vi "Read Stamping.vi"(8 "error in (no error)":errorcluster, 11 "Gluing Procedure in":refnum<class "Gluing Procedure.lvclass">) -> (0 "error out":errorcluster, 2 "Stamping":T1, 3 "Gluing Procedure out":refnum<class "Gluing Procedure.lvclass">)   [LabVIEW 2017, in "Gluing Procedure.lvclass"]
uses:
  Gluing Procedure.lvclass
  Type Definitions/Stamping.ctl
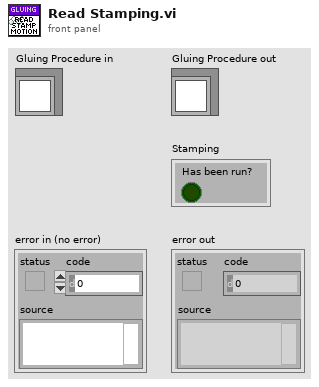
[diagram p1: front panel]
types:
  T1 = typedef "Stamping.ctl" = cluster{"Has been run?":bool}
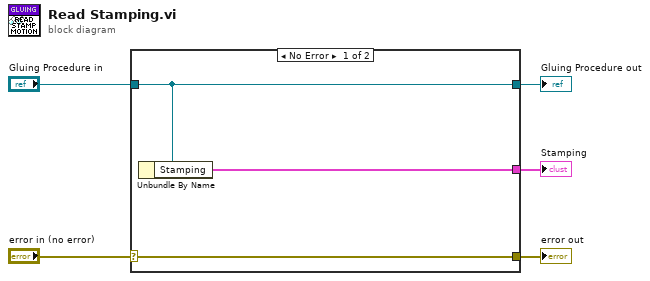
[diagram p0: block diagram]
diagram:
  n1 = case shown="No Error" "error in (no error)" {
    selector: "error in (no error)" -> [w8 w9]
    tunnel: [w8 w9] -> w4
    tunnel: [w7 w10] -> w2
    tunnel: "Gluing Procedure in" -> [w7 w10]
    tunnel: [w6 _] -> w1
    frame No Error {
      n2 = Unbundle By Name(w7) -> ("Stamping"=w6:T1)
    }
    frame Error {
    }
  }
  "error out" <- w4
  "Gluing Procedure out" <- w2
  "Stamping" <- w1
